vi "Autonomous Independent.vi"   [LabVIEW 2014]
doc: "This VI is called when autonomous begins, and will automatically be terminated when autonomous ends. You can carry out timed or sensor driven robot movement independently without needing to return to the caller."
uses:
  Robot Global Data.vi
types:
  T1 = typedef "cluster data.ctl" = cluster{"West Coast Drive Dev-ref":T2, "Driver Gamepad":T12, "Operator Gamepad":T12, "Shifting Solenoid 1":T14, "Motors":cluster{"Lift Motor 1":T3, "Gripper Motor":T3, "Lift Motor 2":T3}, "Limit Switches":cluster{"SwitchDevRef":T16, "SwitchDevRef 2":T16, "SwitchDevRef 3":T16, "SwitchDevRef 4":T16}, "Drive Encoders":cluster{"EncoderDevRef":T19, "EncoderDevRef":T19}, "Gripper Encoder":T19, "Lift Potentiometer":T22, "Shifting Solenoid 2":T14, "Gyro":T25}
  T2 = typedef "WPI_RobotDriveDevRef.ctl" = cluster{"DevStatus":errorcluster, "Motors[]":T3[], "Square Inputs":bool, "Max Output":dbl}
  T3 = typedef "WPI_MotorControlDeviceRef.ctl" = cluster{"DeviceStatus":errorcluster, "Type":T4, "PWM":cluster{"Controller":T5, "PWM Channel":T6, "DeadBand":T7}, "CAN":cluster{"Device Number":u8, "Control Mode":T8, "Semaphore":T9, "Max Vout":dbl, "TalonSRX Control Mode":T10}, "Invert":bool, "TransformRef":T11, "InvTransformRef":T11}
  T4 = typedef "WPI_MotorControlType.ctl" = enum16{"PWM", "CAN", "CANTalonSRX"}
  T5 = typedef "FPGA_TypedefDigitalModule.ctl" = enum16{"Controller 1"}
  T6 = typedef "FPGA_DIOPWMChannel.ctl" = enum8{"PWM 0", "PWM 1", "PWM 2", "PWM 3", "PWM 4", "PWM 5", "PWM 6", "PWM 7", "PWM 8", "PWM 9", "PWM MXP 0", "PWM MXP 1", "PWM MXP 2", "PWM MXP 3", "PWM MXP 4", "PWM MXP 5", "PWM MXP 6", "PWM MXP 7", "PWM MXP 8", "PWM MXP 9", "Invalid"}
  T7 = typedef "WPI_PWMDeadband.ctl" = cluster{"Name":string, "maxPositivePwm":i32, "minPositivePwm":i32, "centerPwm":i32, "maxNegativePwm":i32, "minNegativePwm":i32, "angularRange":u16}
  T8 = typedef "WPI_CANJaguar_ControlMode.ctl" = enum8{"Percent VBus", "Current", "Speed", "Position", "Voltage"}
  T9 = typedef "Semaphore RefNum" = refnum<k1>
  T10 = typedef "WPI_CANTalonSRX_APIControlMode.ctl" = enum8{"Percent VBus", "Speed", "Position", "Slave", "Unchanged / Invalid"}
  T11 = typedef "WPI_PWMTransform_ConPane.ctl" = refnum<vi>
  T12 = typedef "WPI_JoystickDevRef.ctl" = cluster{"Device":T13}
  T13 = typedef "WPI_JoystickDeviceEnum.ctl" = enum16{"USB 0", "USB 1", "USB 2", "USB 3", "USB 4", "USB 5"}
  T14 = typedef "WPI_SolenoidDevRef.ctl" = cluster{"DevStatus":errorcluster, "Pneumatics Control Module":u8, "Forward Solenoid Channel":T15, "Reverse Solenoid Channel":T15}
  T15 = typedef "WPI_SolenoidChannel.ctl" = enum8{"Solenoid 0", "Solenoid 1", "Solenoid 2", "Solenoid 3", "Solenoid 4", "Solenoid 5", "Solenoid 6", "Solenoid 7", "Invalid"}
  T16 = typedef "WPI_SwitchDevRef.ctl" = cluster{"DevStatus":errorcluster, "DIO Channel":T17, "Controller":T5, "CntIndex":T18, "Normally Closed":bool}
  T17 = typedef "FPGA_DIOChannel.ctl" = enum8{"DIO 0", "DIO 1", "DIO 2", "DIO 3", "DIO 4", "DIO 5", "DIO 6", "DIO 7", "DIO 8", "DIO 9", "DIO MXP 0", "DIO MXP 1", "DIO MXP 2", "DIO MXP 3", "DIO MXP 4", "DIO MXP 5", "DIO MXP 6", "DIO MXP 7", "DIO MXP 8", "DIO MXP 9", "DIO MXP 10", "DIO MXP 11", "DIO MXP 12", "DIO MXP 13", "DIO MXP 14", "DIO MXP 15", "Invalid"}
  T18 = typedef "FPGA_CounterCtrSystemIndex.ctl" = enum8{"Ctr 0", "Ctr 1", "Ctr 2", "Ctr 3", "Ctr 4", "Ctr 5", "Ctr 6", "Ctr 7", "Invalid"}
  T19 = typedef "WPI_EncoderDevRef.ctl" = cluster{"DevStatus":errorcluster, "EncoderIndex":T20, "CounterIndex":T18, "DistancePerCount":dbl, "Decoding Type":T21}
  T20 = typedef "FPGA_EncoderIdx.ctl" = enum8{"Enc 0", "Enc 1", "Enc 2", "Enc 3", "Enc 4", "Enc 5", "Enc 6", "Enc 7", "Invalid"}
  T21 = typedef "WPI_EncoderType.ctl" = enum16{"1x", "2x", "4x"}
  T22 = typedef "WPI_PotentiometerDevRef.ctl" = cluster{"DevStatus":errorcluster, "Controller":T23, "Analog Channel":T24, "Invert Output":bool}
  T23 = typedef "FPGA_TypedefAnalogModule.ctl" = enum16{"Controller 1"}
  T24 = typedef "FPGA_AIChannel.ctl" = enum8{"AI 0", "AI 1", "AI 2", "AI 3", "AI MXP 0", "AI MXP 1", "AI MXP 2", "AI MXP 3", "Invalid"}
  T25 = typedef "WPI_GyroDevRef.ctl" = cluster{"DevStatus":errorcluster, "Analog Module":T23, "Analog Channel":T24, "Offset":dbl, "Gain (VoltsPerDegree/Second)":dbl}
  T26 = cluster{"Motors":cluster{"Lift Motor 1":T3, "Gripper Motor":T3, "Lift Motor 2":T3}, "Lift Potentiometer":T22, "Limit Switches":cluster{"SwitchDevRef":T16, "SwitchDevRef 2":T16, "SwitchDevRef 3":T16, "SwitchDevRef 4":T16}, "Gripper Encoder":T19}
  T27 = cluster{"RobotDriveDevRef":T2, "EncoderDevRef":T19, "EncoderDevRef":T19, "GyroDevRef":T25}
  T28 = cluster{"Shifting Solenoid 1":T14, "Shifting Solenoid 2":T14}
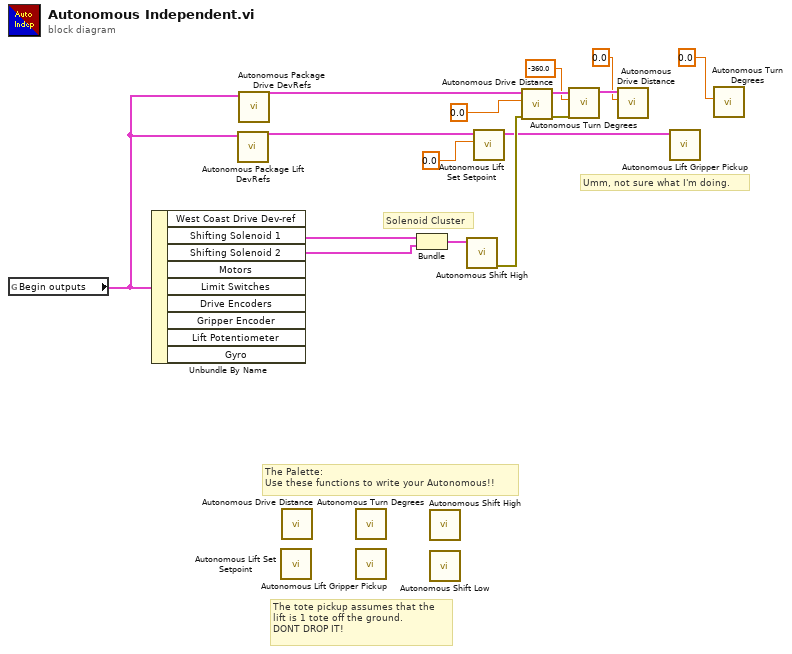
[diagram p0: block diagram]
diagram:
  # "Umm, not sure what I'm doing."
  # "The tote pickup assumes that the \nlift is 1 tote off the ground. \nDONT DROP IT!"
  # "Solenoid Cluster"
  # "The Palette:\nUse these functions to write your Autonomous!!"
  n1 = global read "Robot Global Data.vi" "Begin outputs"() -> (w16:T1)
  n2 = Unbundle By Name(w16) -> ("Shifting Solenoid 1"=w15:T14, "Shifting Solenoid 2"=w14:T14)  [unwired: 7 out]
  n3 = call "Autonomous Package Lift DevRefs.vi"("Begin outputs"=w16) -> ("Lift References"=w3:T26)  [unwired: 9 in, 1 out]
  n4 = call "Autonomous Package Drive DevRefs.vi"("Begin outputs"=w16) -> ("Drive DevRefs"=w12:T27)  [unwired: 9 in, 1 out]
  n5 = call "Autonomous Lift Set Setpoint.vi"() -> ()  [unwired: 10 in, 2 out]
  n6 = call "Autonomous Drive Distance.vi"() -> ()  [unwired: 10 in, 2 out]
  n7 = call "Autonomous Turn Degrees.vi"() -> ()  [unwired: 10 in, 2 out]
  n8 = call "Autonomous Lift Gripper Pickup.vi"() -> ()  [unwired: 10 in, 2 out]
  n9 = Bundle("Shifting Solenoid 1"=w15, "Shifting Solenoid 2"=w14) -> (w13:T28)  [unwired: 1 in]
  n10 = call "Autonomous Shift High.vi"() -> ()  [unwired: 10 in, 2 out]
  n11 = call "Autonomous Shift Low.vi"() -> ()  [unwired: 10 in, 2 out]
  n12 = call "Autonomous Shift High.vi"("Solenoids In"=w13) -> ("error out"=w10:errorcluster)  [unwired: 9 in, 1 out]
  n13 = call "Autonomous Lift Set Setpoint.vi"("Setpoint"=0.0, "Lift References"=w3) -> ("Lift References Out"=w2:T26)  [unwired: 8 in, 1 out]
  n14 = call "Autonomous Drive Distance.vi"("error in (no error)"=w10, "Distance"=0.0, "Drive DevRefs"=w12) -> ("error out"=w9:errorcluster, "drive out"=w8:T27)  [unwired: 7 in]
  n15 = call "Autonomous Turn Degrees.vi"("error in (no error)"=w9, "Angle"=-360.0, "Drive DevRefs"=w8) -> ("Drive DevRefs Out"=w6:T27)  [unwired: 7 in, 1 out]
  n16 = call "Autonomous Drive Distance.vi"("Distance"=0.0, "Drive DevRefs"=w6) -> ()  [unwired: 8 in, 2 out]
  n17 = call "Autonomous Lift Gripper Pickup.vi"("Lift References"=w2) -> ()  [unwired: 9 in, 2 out]
  n18 = call "Autonomous Turn Degrees.vi"("Angle"=0.0) -> ()  [unwired: 9 in, 2 out]
